vi "ATF_Graph_PID_V1.0.vi"() -> ()   [LabVIEW 2022 SP3]
panel:
  out "Vrms DATA MOTOR":dbl(graph)
  out "VIBRATION DATA PUMB":dbl(graph)
  out "Temperature Data":dbl(graph)
  out "RTD DATA PUMB":dbl(graph)
  out "Thermal Graph 3":dbl(graph)
  out "AI_PT&FM DATA PUMB":waveform(dbl)[](graph)
  in  "EXIT":bool
  # "ATF RIG SOFTAWRE"
  # "Version:V1.0"
  # "Release Date:"
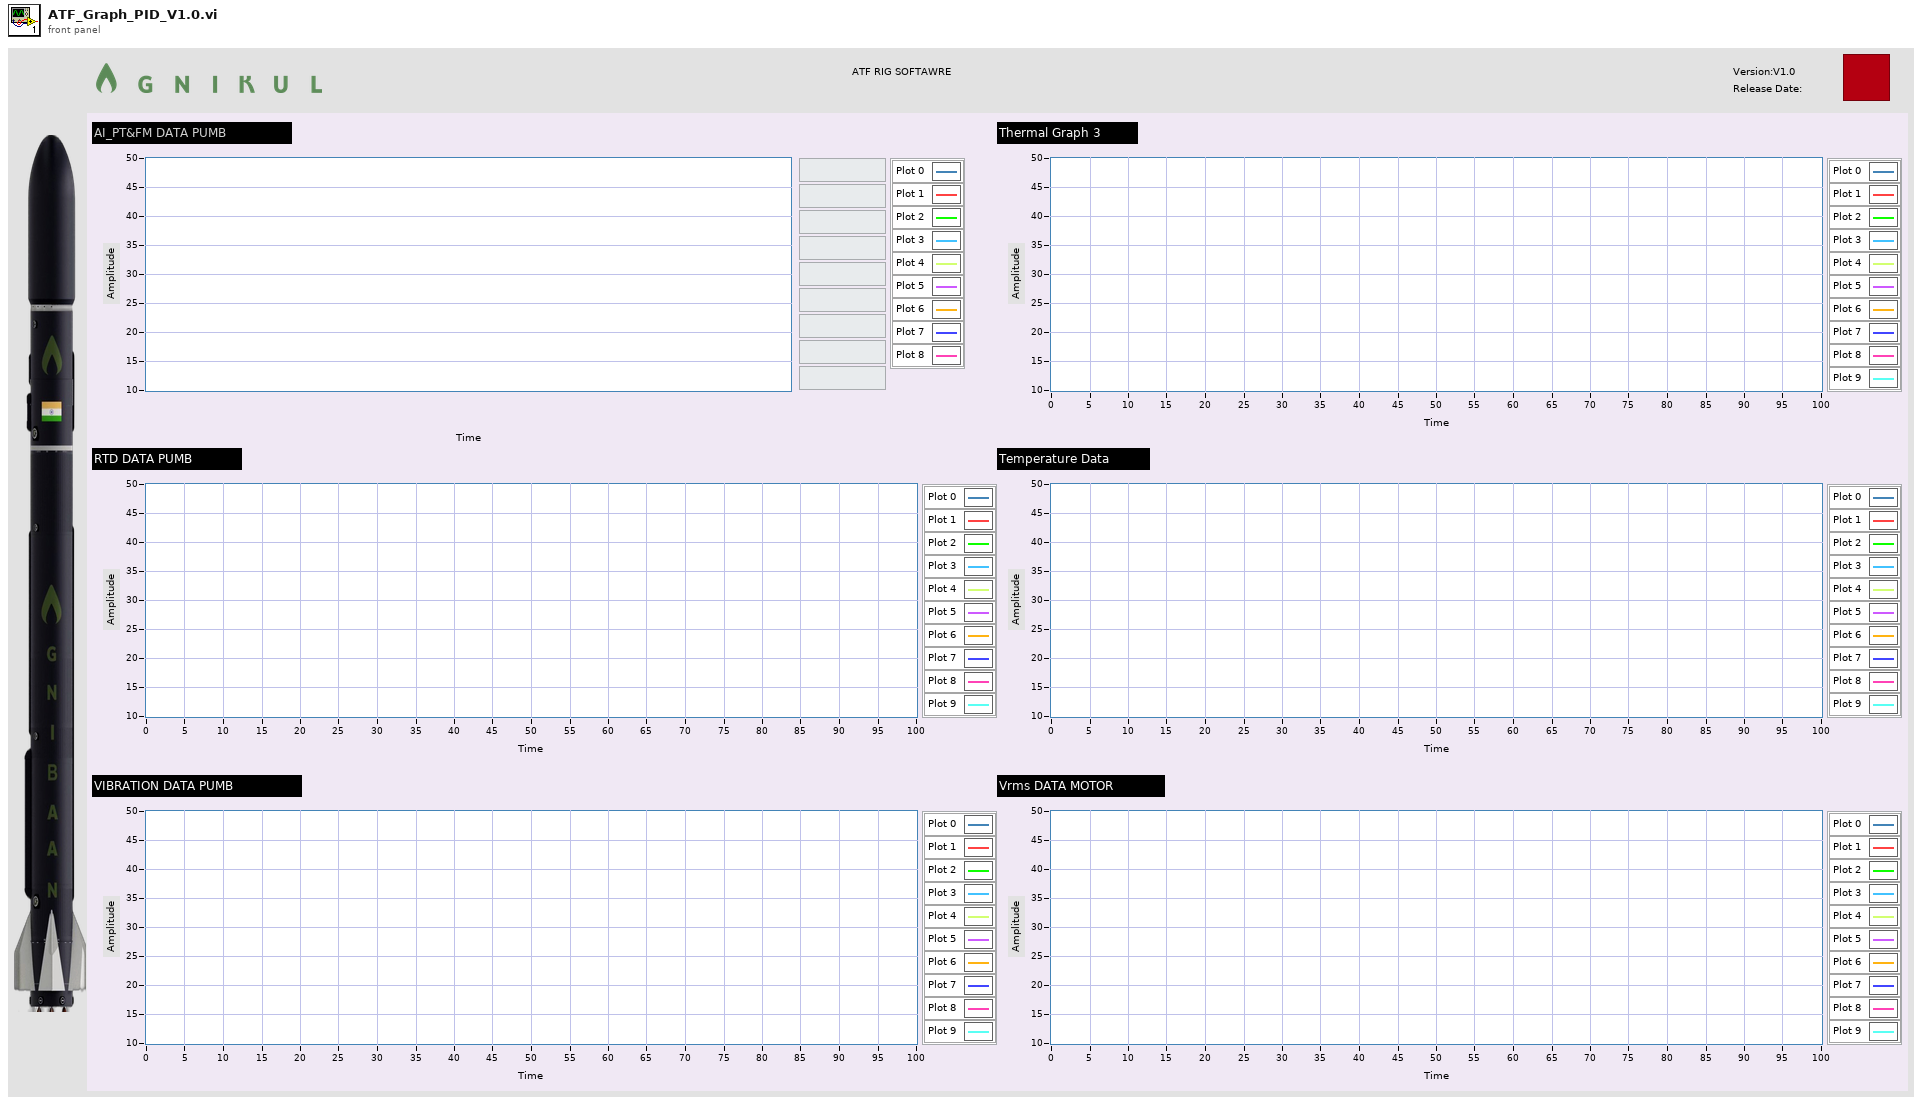
[diagram p1: front panel]
types:
  T1 = cluster{"AI_V_Data":waveform(dbl)[][], "AI_C_Data":waveform(dbl)[][], "AO_Data":waveform(dbl)[][], "DO_Data":waveform(dbl)[][], "DI_Data":digitalwaveform[][], "ACC_Data":waveform(dbl)[][], "TC Data":waveform(dbl)[][], "Drive_A_C":waveform(dbl)[][], "Drive_A_D":waveform(dbl)[][], "Drive_L_C":waveform(dbl)[][], "Drive_L_D":waveform(dbl)[][]}
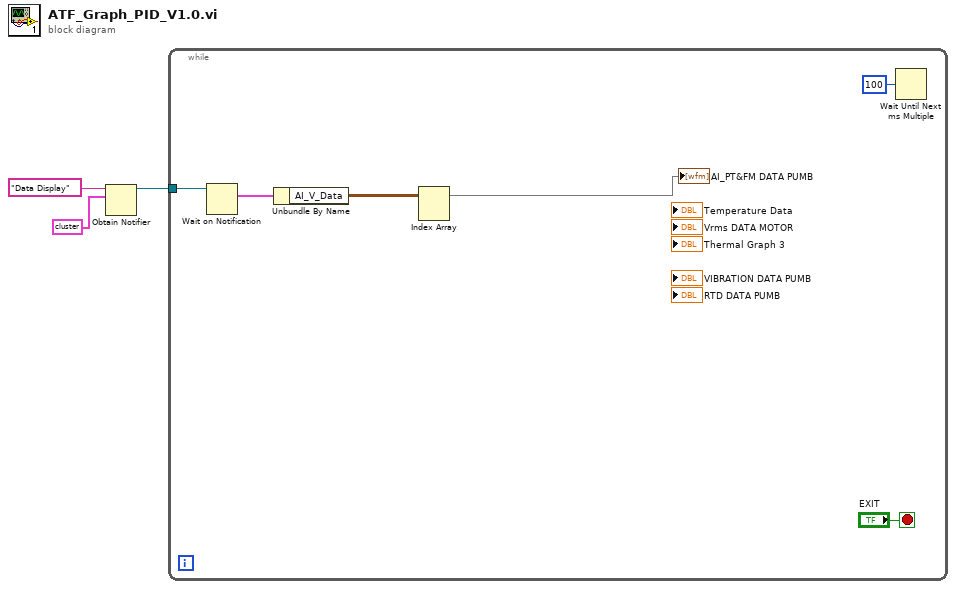
[diagram p0: block diagram]
diagram:
  n1 = Obtain Notifier(name (unnamed)="Data Display", notification data type=T1 data[101848B] ("data out")) -> (notifier out=w1:refnum<notifier>)  [unwired: 2 in, 2 out]
  n2 = while {
    tunnel: w1 -> [w7]
    stop <- "EXIT" stop-if-true
    n3 = Wait on Notification(notifier=w7) -> (notification=w6:T1)  [unwired: 3 in, 3 out]
    n4 = Unbundle By Name(w6) -> ("AI_V_Data"=w5:waveform(dbl)[][])
    n5 = Index Array(array=w5) -> (element=→"AI_PT&FM DATA PUMB":waveform(dbl)[])  [unwired: 2 in]
    n6 = Wait Until Next ms Multiple(millisecond multiple=u32 100) -> ()  [unwired: 1 out]
  }
